vi "CheckThatClassIsWritable.vi"(0 "ClassWriter in":refnum<class "ClassWriter.lvclass">, 1 "Library Refnum":refnum<vi>, 5 "error in (no error)":errorcluster) -> (14 "ClassWriter out":refnum<class "ClassWriter.lvclass">, 19 "error out":errorcluster)   [LabVIEW 2012, in "ClassWriter.lvclass"]
uses:
  <resource>/Framework/Providers/Open_GDS/ClassProviders/Provider_BaseClassInterface/ClassWriter_class/ClassWriter.lvclass
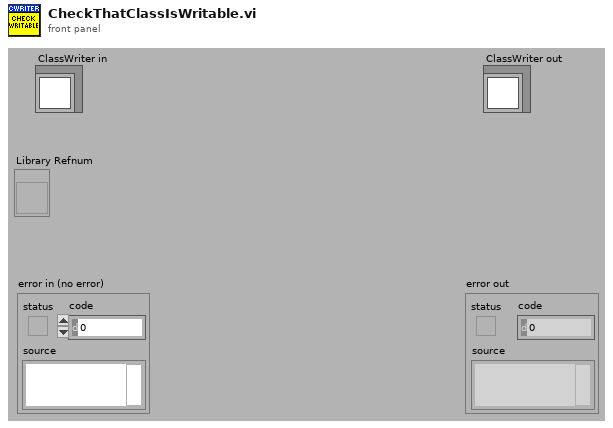
[diagram p1: front panel]
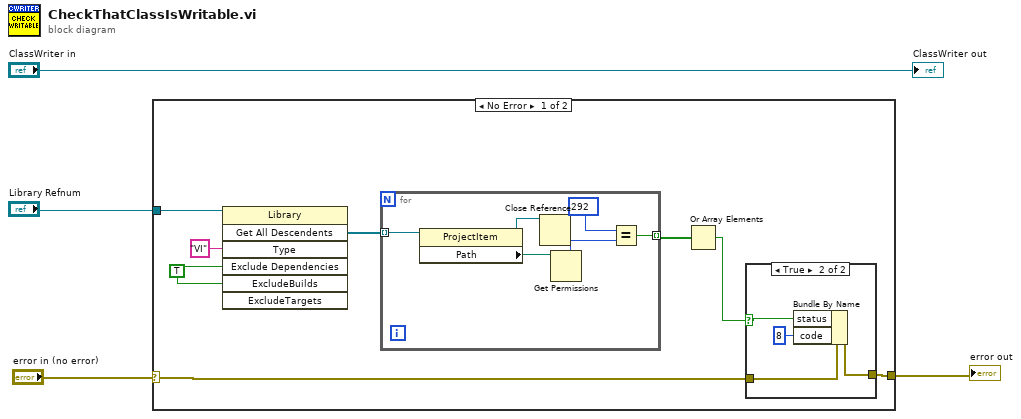
[diagram p0: block diagram]
diagram:
  n1 = case shown="No Error" "error in (no error)" {
    selector: "error in (no error)" -> [w8 w24]
    tunnel: "Library Refnum" -> [w12 _]
    tunnel: [w6 w24] -> w1
    frame No Error {
      w5 = TRUE ("ExcludeDependencies")
      n2 = invoke class="Library" method="Get All Descendents"(reference=w12, "Type"="VI", "Exclude Dependencies"=w5, "ExcludeBuilds"=w5) -> ("All Descendents"=w10:refnum<vi>[])  [unwired: 3 in, 6 out]
      n3 = for {
        tunnel: w10 -> [w23] mode=indexing
        tunnel: [w19] -> w9 mode=indexing
        n4 = property class="ProjectItem"(reference=w23) -> (reference out=w18:refnum<vi>, "Path"=w22:path)  [unwired: 1 in, 1 out]
        n5 = Close Reference(reference=w18) -> ()  [unwired: 1 in, 1 out]
        n6 = Get Permissions(11:w22) -> (5:w21:i16)  [unwired: 1 in, 4 out]
        n7 = Equal?(x=i16 292, y=w21) -> (x = y?=w19:bool)
      }
      n8 = Or Array Elements(Boolean array=w9) -> (logical OR=w7:bool)
      n9 = case shown="True" w7 {
        selector: w7 -> [_ w15]
        tunnel: w8 -> [w13 w17]
        tunnel: [w13 w16] -> w6
        frame False {
        }
        frame True {
          n10 = Bundle By Name(cluster=w17, "status"=w15, "code"=8) -> (w16:errorcluster)
        }
      }
    }
    frame Error {
    }
  }
  "error out" <- w1
  "ClassWriter out" <- "ClassWriter in"
